vi "Reverse_Motor_Direction.vi"(10 "Numeric":u16) -> (2 "Numeric 2":u16)   [LabVIEW 2013, in "ProcessorHelperFunctions.lvlib"]
uses:
  ProcessorHelperFunctions.lvlib
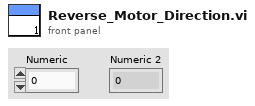
[diagram p1: front panel]
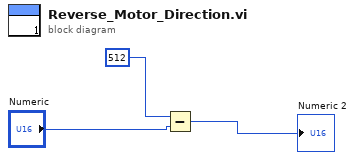
[diagram p0: block diagram]
diagram:
  n1 = Subtract(x=u16 512, y="Numeric") -> (x-y=→"Numeric 2":u16)
